vi "AB_Log_Open.vi"(8 "error in (no error)":errorcluster, 9 "build spec name":string, 11 "Objects":T1[](array[typedef])) -> (0 "error out":errorcluster)   [LabVIEW 2020]
uses:
  <resource>/Framework/Providers/API/ItemRef.ctl
  <vilib>/AppBuilder/logging/AB_Log_File_Action.ctl
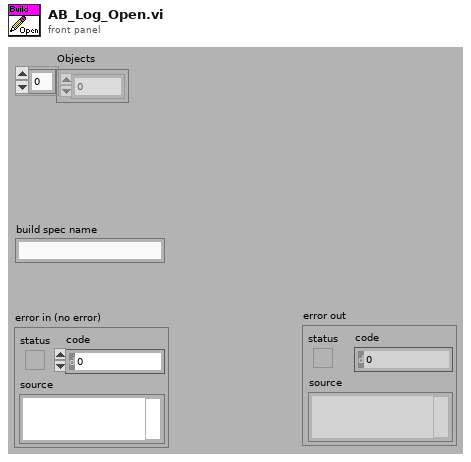
[diagram p1: front panel]
types:
  T1 = typedef "ItemRef.ctl" = u64
  T2 = typedef "AB_Log_File_Action.ctl" = enum16{"write", "open", "close"}
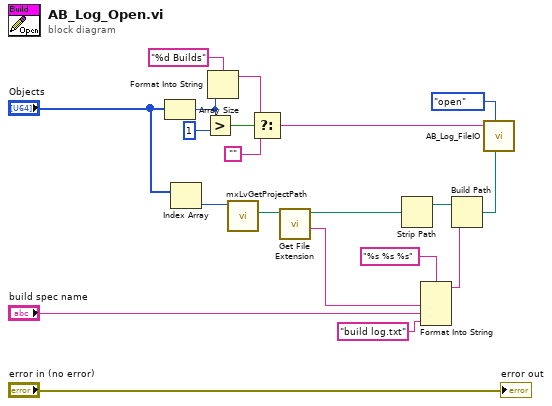
[diagram p0: block diagram]
diagram:
  n1 = Array Size(array="Objects") -> (size(s)=w15:i32)
  n2 = Index Array(array="Objects") -> (element=w7:T1)  [unwired: 1 in]
  n3 = Greater?(x=w15, y=1) -> (0:w17:bool)
  n4 = Format Into String(format string="%d Builds", w15) -> (resulting string=w14:string)  [unwired: 2 in, 1 out]
  n5 = call <resource>:"mxLvGetProjectPath.vi"("Item"=w7) -> ("Project Path"=w6:path)  [unwired: 8 in, 2 out]
  n6 = Select(t=w14, s=w17, f="") -> (s? t:f=w8:string)
  n7 = call <vilib>:"Get File Extension.vi"("file"=w6) -> ("filename without extension"=w3:string, "dup file"=w11:path)  [unwired: 6 in, 3 out]
  n8 = Strip Path(path=w11) -> (stripped path=w10:path)  [unwired: 1 out]
  n9 = Format Into String(format string="%s %s %s", w3, "build spec name", "build log.txt" ("string")) -> (resulting string=w4:string)  [unwired: 2 in, 1 out]
  n10 = Build Path(base path=w10, name or relative path=w4) -> (appended path=w9:path)
  n11 = call <vilib>:"AB_Log_FileIO.vi"("file"=w9, "fileAction"=AB_Log_File_Action."open", "newSection"=w8) -> ()  [unwired: 8 in, 1 out]
  "error out" <- "error in (no error)"
